vi "StringToArrayFloat.vi"(8 "entrée d'erreur (pas d'erreur)":errorcluster, 11 "Return value":string) -> (0 "error IO":errorcluster, 2 "2DArray":dbl[][](array[numeric]), 3 "1DArray":dbl[](array[numeric]))   [LabVIEW 2020]
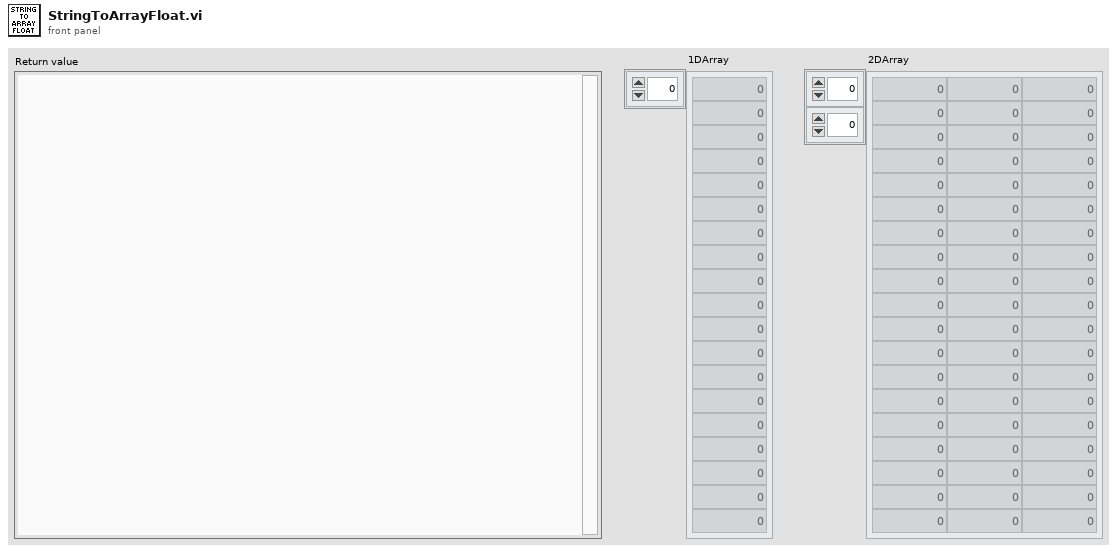
[diagram p1: front panel]
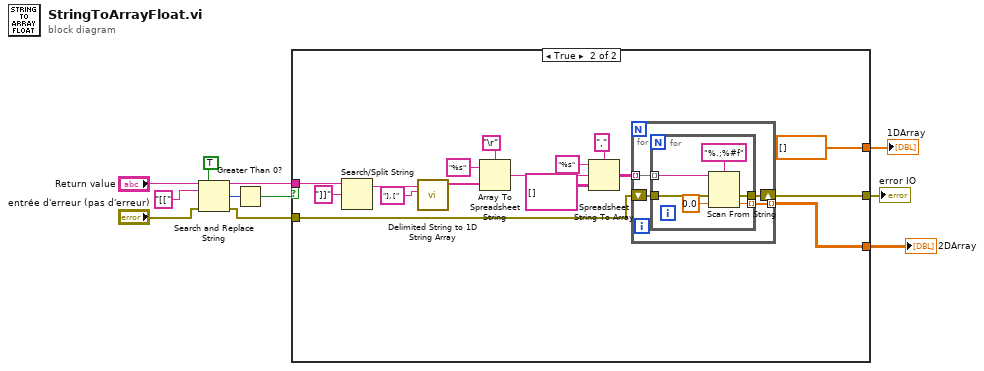
[diagram p0: block diagram]
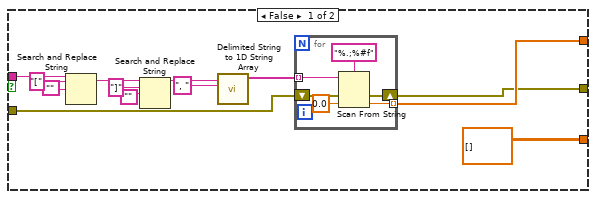
[diagram p2: hidden frame]
diagram:
  n1 = Search and Replace String(replace all?=TRUE ("replace all? (F)"), input string="Return value", search string="[[", error in="entrée d'erreur (pas d'erreur)") -> (result string=w6:string, number of replacements=w8:i32, error out=w3:errorcluster)  [unwired: 4 in, 1 out]
  n2 = Greater Than 0?(x=w8) -> (x > 0?=w7:bool)
  n3 = case shown="True" w7 {
    tunnel: [dbl[][] [] w33] -> w11
    tunnel: w6 -> [w15 w42]
    tunnel: [w22 dbl[] []] -> w5
    tunnel: w3 -> [w13 w32]
    tunnel: [w12 w31] -> w2
    frame False {
      n4 = Search and Replace String(input string=w15, search string="[", replace string="") -> (result string=w16:string)  [unwired: 5 in, 3 out]
      n5 = Search and Replace String(input string=w16, search string="]", replace string="") -> (result string=w14:string)  [unwired: 5 in, 3 out]
      n6 = call <vilib>:"Delimited String to 1D String Array.vi"("delimiter"=", ", "delimited string"=w14) -> ("string array"=w24:string[])  [unwired: 9 in]
      n7 = for {
        tunnel: w24 -> [w28] mode=indexing
        tunnel: [w27] -> w22 mode=indexing
        shift-right: [w25] -> w12
        shift-left: w13 -> [w26]
        n8 = Scan From String(format string="%.;%#f", input string=w28, error in=w26, default 1=0.0 ("default value 1")) -> (error out=w25:errorcluster, output 1=w27:dbl)  [unwired: 1 in, 2 out]
      }
    }
    frame True {
      n9 = Search/Split String(string=w42, search string/char (-)="]]" ("chaîne/car. recherché (-)")) -> (substring before match=w41:string)  [unwired: 1 in, 2 out]
      n10 = call <vilib>:"Delimited String to 1D String Array.vi"("delimiter"="], [", "delimited string"=w41) -> ("string array"=w44:string[])  [unwired: 9 in]
      n11 = Array To Spreadsheet String(delimiter (Tab)="\r", array=w44, 3:"%s" ("chaîne de format")) -> (spreadsheet string=w35:string)
      n12 = Spreadsheet String To Array(delimiter (Tab)="," ("séparateur (Tabulation)"), format string="%s" ("chaîne de format"), spreadsheet string=w35, array type (2D Dbl)=string[][] []) -> (array=w34:string[][])
      n13 = for {
        tunnel: [w50] -> w33 mode=indexing
        tunnel: w34 -> [w49] mode=indexing
        shift-right: [w47] -> w31
        shift-left: w32 -> [w48]
        n14 = for {
          tunnel: [w54] -> w50 mode=indexing
          tunnel: w49 -> [w53] mode=indexing
          tunnel: w48 -> [w52]
          tunnel: [w51] -> w47
          n15 = Scan From String(format string="%.;%#f", input string=w53, error in=w52, default 1=0.0 ("default value 1")) -> (error out=w51:errorcluster, output 1=w54:dbl)  [unwired: 1 in, 2 out]
        }
      }
    }
  }
  "2DArray" <- w11
  "1DArray" <- w5
  "error IO" <- w2
